vi "1D String Array to Delimited String.vi"(10 "delimiter":string="\t", 11 "string array":string[](array[string])) -> (3 "delimited string":string)   [LabVIEW 2017]
doc: "Converts the elements of a one-dimensional string array to a single string with input array elements separated by a delimiting character."
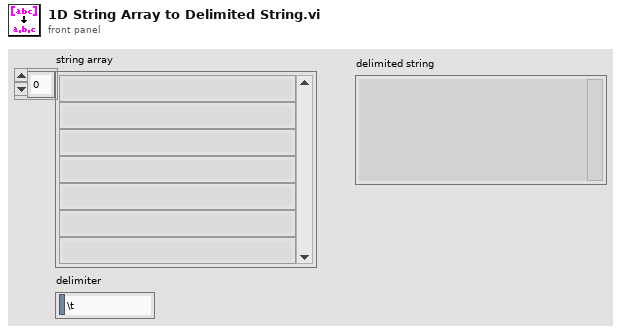
[diagram p1: front panel]
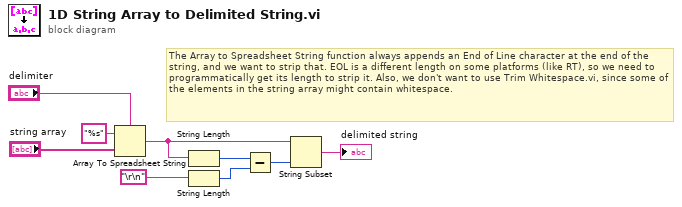
[diagram p0: block diagram]
diagram:
  # "The Array to Spreadsheet String function always appends an End of Line character at the end of the string, and we want to strip that. EOL is a different length on some platforms (like RT), so we need to programmatically get its length to strip it. Also, we don't want to use Trim Whitespace.vi, since some of the elements in the string array might contain whitespace."
  n1 = Array To Spreadsheet String(delimiter (Tab)="delimiter", array="string array", 3:"%s" ("format string")) -> (spreadsheet string=w3:string)
  n2 = String Length(string=w3) -> (length=w5:i32)
  n3 = String Length(string="\r\n") -> (length=w4:i32)
  n4 = Subtract(x=w5, y=w4) -> (x-y=w2:i32)
  n5 = String Subset(string=w3, length (rest)=w2) -> (substring=→"delimited string":string)  [unwired: 1 in]
